vi "panel_hardware_resource_checkout.vi"(8 "error in (no error)":errorcluster, 9 "panel_number":T1, 10 "Self?":bool=TRUE, 11 "panel in":refnum<class "panel.lvclass">) -> (0 "error out":errorcluster, 1 "timed out?":bool, 2 "hardware.lvclass":refnum<class "hardware.lvclass">, 3 "panel out":refnum<class "panel.lvclass">)   [LabVIEW 2015, in "panel.lvclass"]
uses:
  panel.lvclass
  Hardware Class/hardware/hardware.lvclass
  front_panel_class/hardware_caller_queue_numbers.ctl
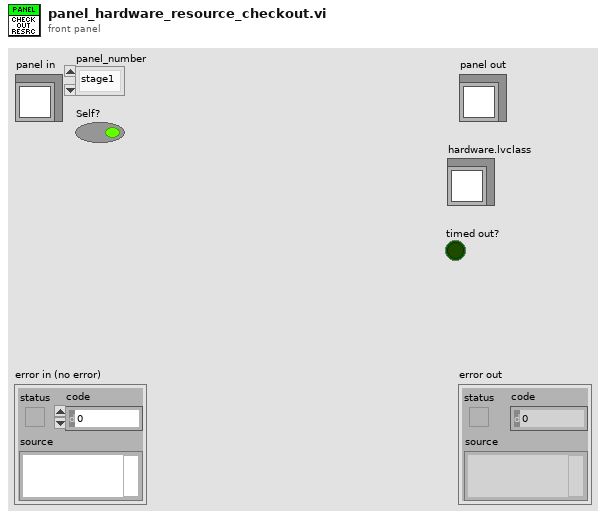
[diagram p1: front panel]
types:
  T1 = typedef "hardware_caller_queue_numbers.ctl" = enum16{"stage1", "stage2", "experiment", "detector"}
  T2 = typedef "hardware_seqs.ctl" = refnum<queue>[]
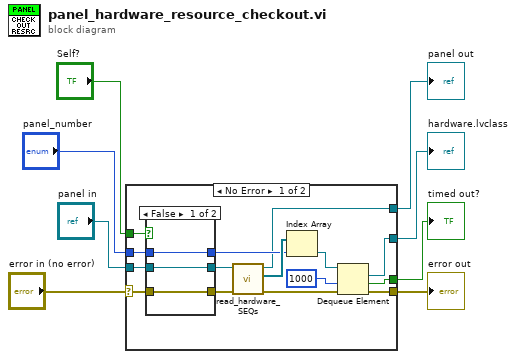
[diagram p0: block diagram]
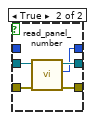
[diagram p2: hidden frame]
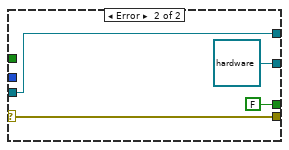
[diagram p3: hidden frame]
diagram:
  n1 = case shown="No Error" "error in (no error)" {
    selector: "error in (no error)" -> [w23 w35]
    tunnel: [w11 w35] -> w3
    tunnel: [w12 w34] -> w6
    tunnel: "panel in" -> [w21 w34]
    tunnel: [w14 refnum<class "hardware.lvclass"> refnum ("hardware.lvclass")] -> w5
    tunnel: [w13 FALSE ("timed out?")] -> w4
    tunnel: "Self?" -> [w10 _]
    tunnel: "panel_number" -> [w9 _]
    frame No Error {
      n2 = case shown="False" w10 {
        tunnel: w23 -> [w24 w31]
        tunnel: [w24 w30] -> w22
        tunnel: w21 -> [w25 w29]
        tunnel: [w25 w28] -> w20
        tunnel: [w26 w27] -> w18
        tunnel: w9 -> [w26 _]
        frame False {
        }
        frame True {
          n3 = call "read_panel_number.vi"("error in (no error)"=w31, "panel in"=w29) -> ("error out"=w30:errorcluster, "panel_number"=w27:T1, "panel out"=w28:refnum<class "panel.lvclass">)  [unwired: 7 in]
        }
      }
      n4 = call "read_hardware_SEQs.vi"("error in (no error)"=w22, "panel in"=w20) -> ("error out"=w15:errorcluster, "hardware_SEQs"=w19:T2, "panel out"=w12:refnum<class "panel.lvclass">)  [unwired: 7 in]
      n5 = Index Array(array=w19, index=w18) -> (element=w17:refnum<queue>)
      n6 = Dequeue Element(queue=w17, timeout in ms (-1)=1000, error in (no error)=w15) -> (element=w14:refnum<class "hardware.lvclass">, timed out?=w13:bool, error out=w11:errorcluster)  [unwired: 1 out]
    }
    frame Error {
    }
  }
  "error out" <- w3
  "panel out" <- w6
  "hardware.lvclass" <- w5
  "timed out?" <- w4
